vi "VCS Get Max Following Error.vi"(8 "error in (no error)":errorcluster, 11 "axis in":cluster{"keyHandle":u32, "nodeId":u16}={"keyHandle"=0, "nodeId"=1}) -> (0 "error out":errorcluster, 1 "maxFollowingError":u32, 3 "axis out":cluster{"keyHandle":u32, "nodeId":u16}={"keyHandle"=0, "nodeId"=1})   [LabVIEW 2019, in "maxonEPOS.lvlib"]
doc: "<B>VCS_GetMaxFollowingError</B>reads the maximal allowed following error parameter."
uses:
  Examples/maxonEPOS.lvlib
  Resources/EposCmd.dll
  Resources/EposCmd64.dll
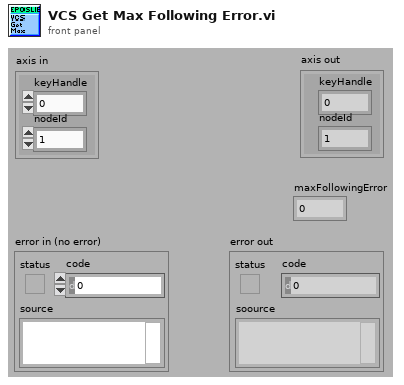
[diagram p1: front panel]
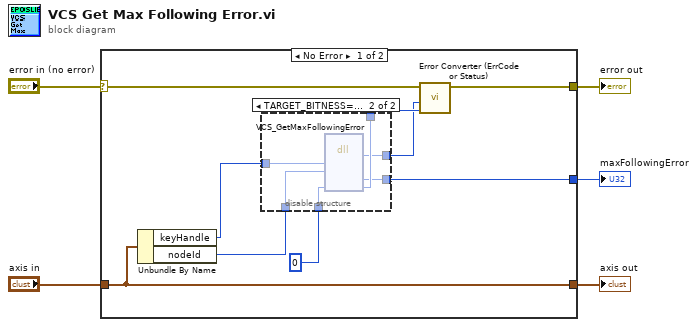
[diagram p0: block diagram]
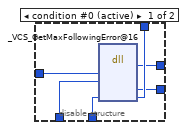
[diagram p2: hidden frame]
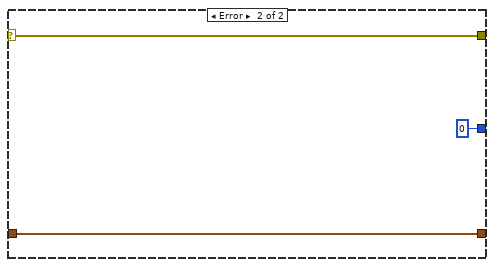
[diagram p3: hidden frame]
diagram:
  n1 = case shown="No Error" "error in (no error)" {
    selector: "error in (no error)" -> [w12 w28]
    tunnel: "axis in" -> [w14 w29]
    tunnel: [w14 w29] -> w4
    tunnel: [w13 w28] -> w3
    tunnel: [w6 u32 0 ("pMaxFollowingError")] -> w1
    frame No Error {
      n2 = Unbundle By Name(w14) -> ("keyHandle"=w11:u32, "nodeId"=w10:u16)
      n3 = disable-structure shown="TARGET_BITNESS==64" {
        disable-tunnel: w11 -> [w20 w26]
        disable-tunnel: w10 -> [w19 w25]
        disable-tunnel: u32 0 ("pErrorCode") -> [w18 w24]
        disable-tunnel: [w17 w23] -> w8
        disable-tunnel: [w16 w22] -> w7
        disable-tunnel: [w15 w21] -> w6
        frame condition #0 (active) {
          n4 = dll-call lib="C:/workspace/project/scancon/sw/SSI_Tool/InstrumentsInterfaces/Motordriver/maxon EPOS/Resources/EposCmd.*" fn="_VCS_GetMaxFollowingError@16"("KeyHandle"=w20, "NodeId"=w19, "pErrorCode"=w18) -> (w16:i32, "pMaxFollowingError"=w15:u32, "pErrorCode"=w17:u32)  [unwired: 6 in, 2 out]
        }
        frame condition #1 {
          n5 = dll-call lib="C:/setup/Resources/EposCmd64.*" fn="VCS_GetMaxFollowingError" ("EposCmd.dll:_VCS_GetMaxFollowingError@16")("KeyHandle"=w26, "NodeId"=w25, "pErrorCode"=w24) -> ("Rückgabetyp"=w22:i32, "pMaxFollowingError"=w21:u32, "pErrorCode"=w23:u32)  [unwired: 6 in, 2 out]
        }
      }
      n6 = call "Error Converter (ErrCode or Status).vi"("error code"=w8, "return type"=w7, "error in (no error)"=w12) -> ("error out"=w13:errorcluster)  [unwired: 7 in]
    }
    frame Error {
    }
  }
  "maxFollowingError" <- w1
  "error out" <- w3
  "axis out" <- w4
